vi "10-Tap 8-bit Camera without DRAM (FPGA-SIM)RandomSimDataNoHostDMAsNoAnalysis.vi"() -> ()   [LabVIEW 2013]
doc: "This is the FPGA VI for the 10-Tap 8-Bit Camera with DRAM example. This example demonstrates how to acquire images from a 10-tap, 8-bit, extended configuration, Camera Link camera and transfer the images to the host. This example supports area scan and line scan cameras for both continuous and finite acquisitions.\n\nThis example also demonstrates the use of DRAM as a frame buffer for very high speed acquisitions. Data packing and flow-control are also employed to maximize use of the available DRAM and FIFOs in terms of both memory space and performance.\n\nAdditionally, the example demonstrates the serial server, which allows third-party camera configuration utilities to communicate with the camera using the Camera Link serial interface while this VI is running."
uses:
  <vilib>/rvi/DataTransferAndStorage/Container/XNode/niFpgaContainer.xnode
  <vilib>/Platform/TimedLoop/XDataNode/XDataNode.xnode
  <vilib>/Platform/TimedLoop/XDataNode/timing_clust.ctl
  <vilib>/Platform/TimedLoop/XDataNode/XDNodeRunTimeDep.lvlib
  <vilib>/Platform/TimedLoop/XDataNode/wakeup.ctl
  <vilib>/Platform/TimedLoop/XDataNode/nitl_modes.ctl
  <vilib>/rvi/FIFO/Fifo_Resource/nirvififoEmulationRead.vi
  <vilib>/rvi/FIFO/Fifo_Resource/nirvififoEmulationWrite.vi
  FPGA/Globals/Accumulated Sector Intensity.vi
  FPGA/Globals/Pixel Location Global.vi
  FPGA/Globals/Wing Square Wave Frequency Global.vi
  FPGA/Globals/Sector Parameter Global.vi
  <vilib>/rvi/FIFO/Fifo_Resource/nirvififoEmulationGetNumberOfElementsToWrite.vi
  <vilib>/rvi/FIFO/Fifo_Resource/nirvififoEmulationGetNumberOfElementsToRead.vi
  Common/CL Signal Mapping.ctl
  Common/CL Configuration.ctl
  FPGA/Sector/Accumulate/Sector Parameter Cluster.ctl
panel:
  in  "Sim Data":u64=44
  out "Number of Elements to Write Sector Grouping FIFO":u32
  out "Accumulate Ticks":u32
  out "Analysis Ticks":u32
  out "Target Sim TO":bool
  out "Cam Data Timeout":bool
  out "Sector FIFO Timeout":bool
  out "Host DMA Timeout":bool
  out "Number of Elements to Read Cam Data":u32
  out "Number of Elements to Write Host DMA":u32
  in  "Words per image":u32=1000
  in  "Y Resolution":u16=1000
  in  "X Resolution":u16=1000
  in  "[Average BG Intensity]":u8[](array[numeric])=[0, 0, 0, 0, 0, 0, 0, 0, 0, 0, 0, 0, 0, 0, 0, 0, 0, 0, 0, 0, 0, 0, 0, 0, 0, 0, 0, 0, 0, 0, 0, 0]
  in  "Sector Threshold":u8
  in  "# of Frames to Average":u8=1
  in  "Sector Parameters Right":T1={"Start Angle"=0.0, "End Angle"=0.4708251953125, "Inner Radius"=309, "Outter Radius"=405, "Hinge X"=685, "Hinge Y"=527, "NumWingSectors"=8}
  in  "Sector Parameters Left":T1={"Start Angle"=0.65740966796875, "End Angle"=0.99468994140625, "Inner Radius"=309, "Outter Radius"=405, "Hinge X"=464, "Hinge Y"=534, "NumWingSectors"=8}
  in  "CL Config.Configuration":T2=enum."Full"
  in  "CL Config.Signal Mapping":T3=enum."Basler 10-tap"
  in  "CL Config.Line Scan":bool
  in  "CL Config.DVAL Active High":bool=TRUE
  in  "CL Config.LVAL Active High":bool=TRUE
  in  "CL Config.FVAL Active High":bool=TRUE
  in  "CL Config.Spare Active High":bool=TRUE
  in  "Acq Control.Line Scan Height":u32
  in  "Acq Control.Frames To Acq":u32
  in  "Acq Control.Acquire":bool
  in  "Acq Control.Cancel Acq":bool
  in  "Acq Control.Ignore DVAL":bool
  in  "Acq Control.Initialize":bool
  out "Acq Status.Acq In Progress":bool
  out "Acq Status.Clocks Per Line":u32
  out "Acq Status.Frames Acq'd":u32
  out "Acq Status.Lines Per Frame":u32
  out "Acq Status.DMA Write Timeout":bool
  out "Acq Status.Initialized":bool
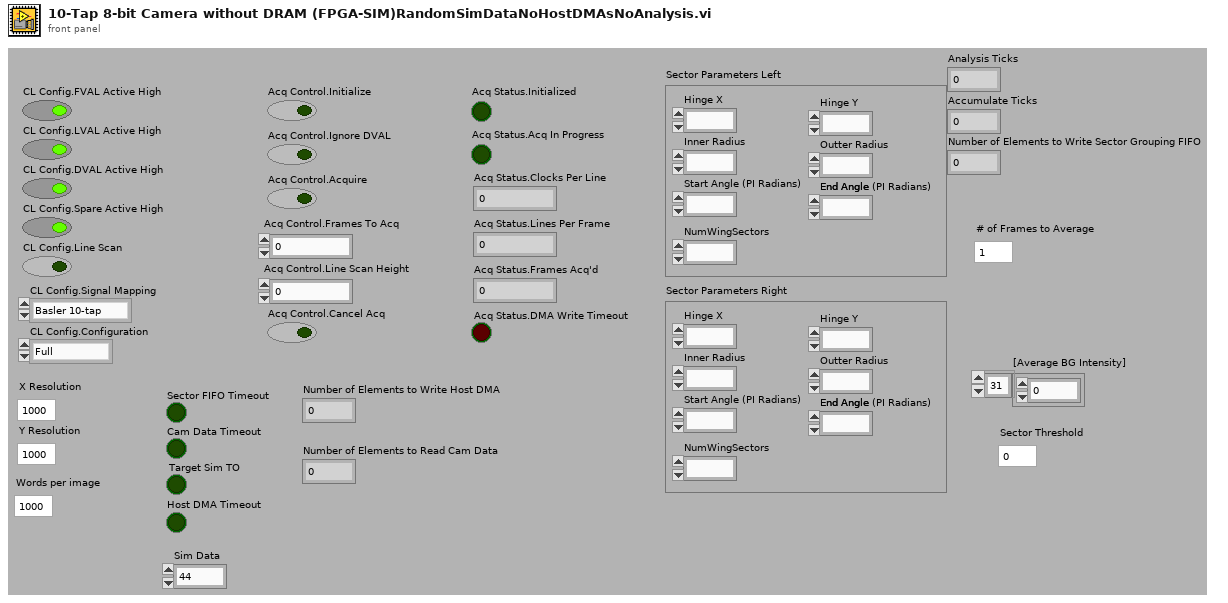
[diagram p1: front panel]
types:
  T1 = typedef "Sector Parameter Cluster.ctl" = cluster{"Start Angle":fxp<+/-,17,2>, "End Angle":fxp<+,17,3>, "Inner Radius":u16, "Outter Radius":u16, "Hinge X":u16, "Hinge Y":u16, "NumWingSectors":u8}
  T2 = typedef "CL Configuration.ctl" = enum8{"Base", "Medium", "Full"}
  T3 = typedef "CL Signal Mapping.ctl" = enum8{"Standard", "Basler 10-tap", "Vosskühler 10-tap"}
  T4 = typedef "XDNodeRunTimeDep.lvlib/timing_clust.ctl" = cluster{"Expected End [f-1]":u64, "Actual End [f-1]":u64, "Finished Late? [f-1]":bool, "Expected End [i-1]":u64, "Actual End [i-1]":u64, "Finished Late? [i-1]":bool, "Expected Start [i]":u64, "Actual Start [i]":u64, "Expected Start [f]":u64, "Actual Start [f]":u64, "Source Name":string, "Structure Name":string, "Period":i64, "Deadline":i64, "Offset":i64, "Start":i64, "Priority":i32, "Timeout":i32, "Mode":T5, "Wakeup Reason":T6, "Error":errorcluster, "Source Type":string, "Secondary Source Type":string, "Global End Time":u64, "Global Start Time":u64, "Frame Duration":u64, "Iteration Duration":u64, "Assigned CPU":i32, "I/O Scan Engine Mode":u32}
  T5 = typedef "XDNodeRunTimeDep.lvlib/nitl_modes.ctl" = enum32{"No Change", "Process missed periods, maintain original phase", "Discard missed periods, maintain original phase", "Process missed periods, ignore original phase", "Discard missed periods, ignore original phase"}
  T6 = typedef "XDNodeRunTimeDep.lvlib/wakeup.ctl" = enum32{"Normal", "Aborted", "Asynchronous wakeup", "Timing source error", "Timed loop error", "Timeout"}
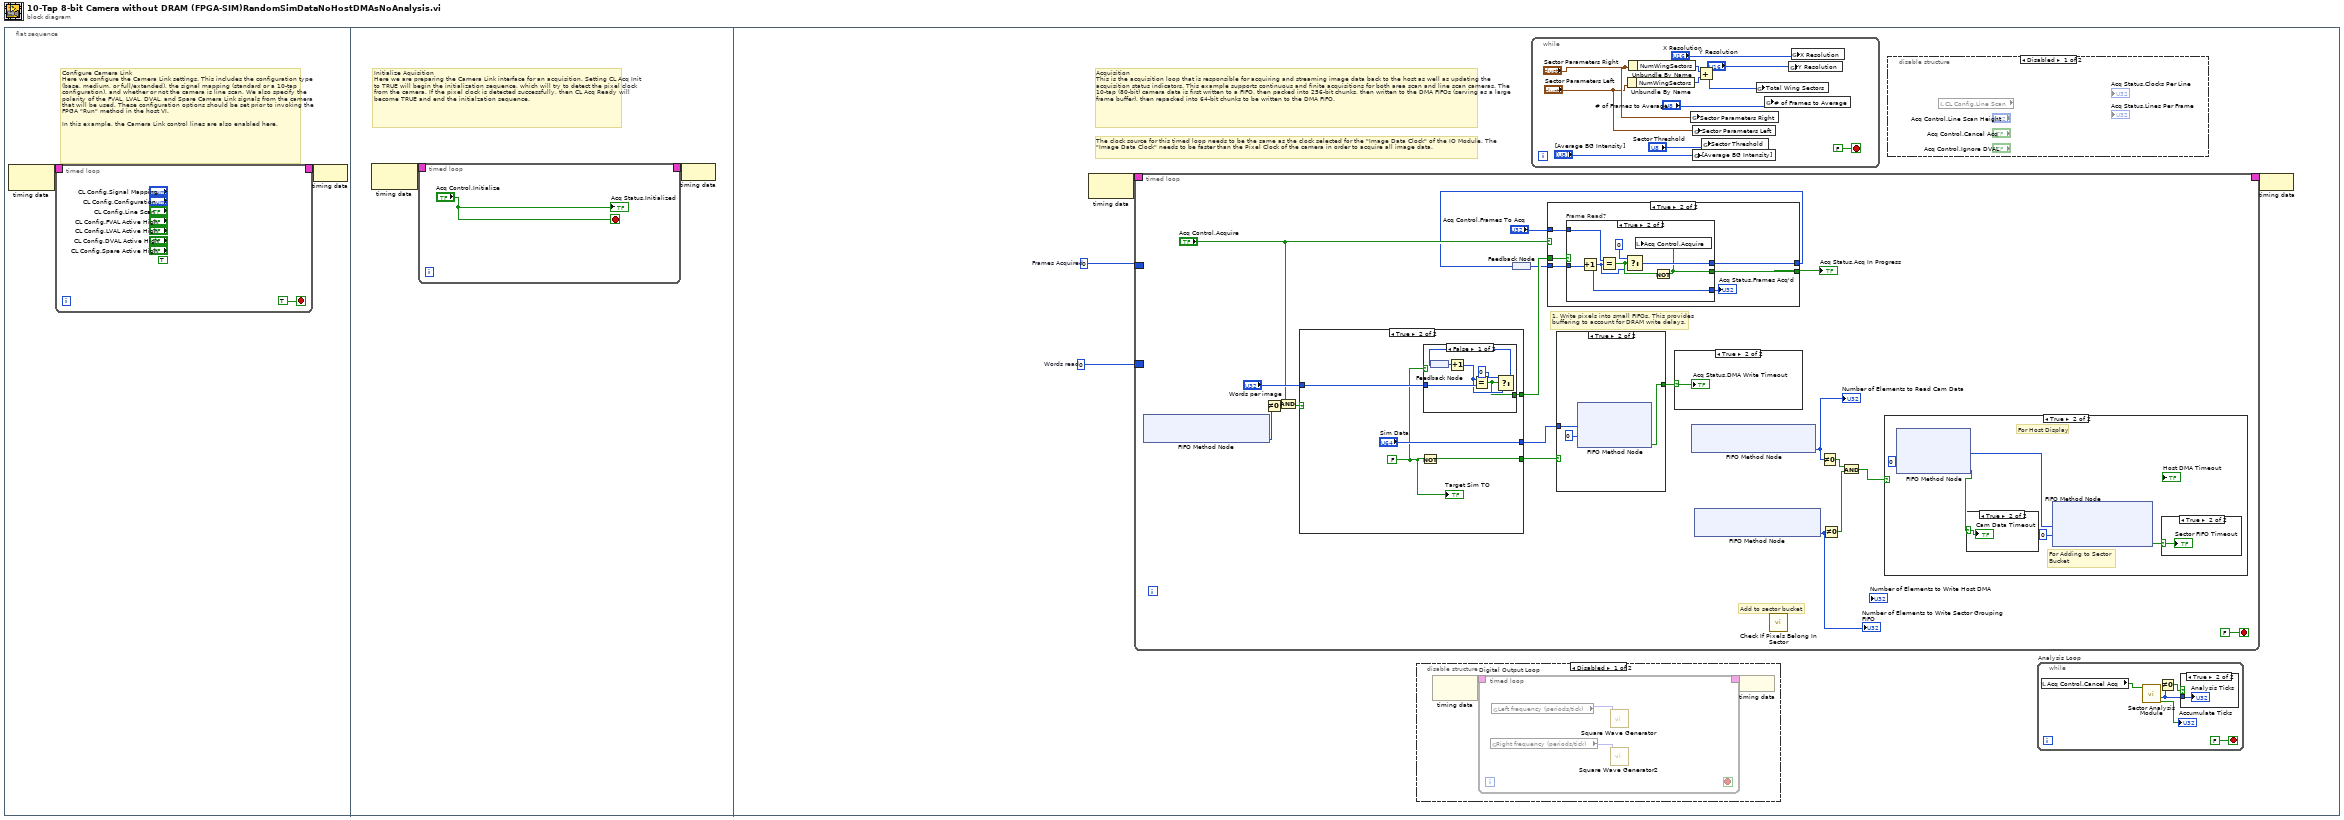
[diagram p0: block diagram]
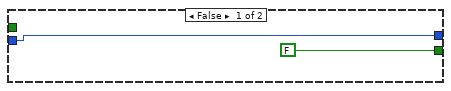
[diagram p6: hidden frame]
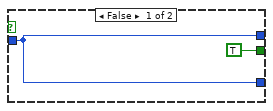
[diagram p7: hidden frame]
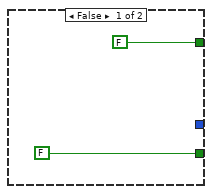
[diagram p8: hidden frame]
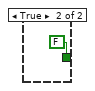
[diagram p9: hidden frame]
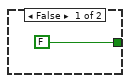
[diagram p13: hidden frame]
diagram:
  n1 = flat-sequence {
    frame #0 {
      # "Configure Camera Link\nHere we configure the Camera Link settings. This includes the configuration type (base, medium, or full/extended), the signal mapping (standard or a 10-tap configuration), and whether or not the camera is line scan. We also specify the polarity of the FVAL, LVAL, DVAL, and Spare Camera Link signals from the camera that will be used. These configuration options should be set prior to invoking the FPGA \"Run\" method in the host VI.\n\nIn this example, the Camera Link control lines are also enabled here."
      n2 = node-c288() -> (w2:T4)  [unwired: 1 in]
      n3 = timed-loop {
        timing: w2 -> [_]
        timing-out: [_] -> w1
        stop <- TRUE stop-if-true
        (unwired) TRUE ("IO Module\\CL Control Enable")
      }
      n4 = node-c288(w1) -> ()
    }
    frame #1 {
      # "Initialize Aquisition\nHere we are preparing the Camera Link interface for an acquisition. Setting CL Acq Init to TRUE will begin the initialization sequence, which will try to detect the pixel clock from the camera. If the pixel clock is detected successfully, then CL Acq Ready will become TRUE and end the initialzation sequence."
      n5 = node-c288() -> (w9:T4)  [unwired: 1 out]
      n6 = timed-loop {
        timing: w9 -> [_]
        timing-out: [_] -> w8
        stop <- "Acq Control.Initialize" stop-if-true
        "Acq Status.Initialized" <- "Acq Control.Initialize"
      }
      n7 = node-c288(w8) -> ()
    }
    frame #2 {
      w15 = u32 0  # Frames Acquired
      w16 = u32 0  # Words read
      # "The clock source for this timed loop needs to be the same as the clock selected for the \"Image Data Clock\" of the IO Module. The \"Image Data Clock\" needs to be faster than the Pixel Clock of the camera in order to acquire all image data."
      # "Acquisition\nThis is the acquisition loop that is responsible for acquiring and streaming image data back to the host as well as updating the acquisition status indicators. This example supports continuous and finite acquisitions for both area scan and line scan cameras. The 10-tap (80-bit) camera data is first written to a FIFO, then packed into 256-bit chunks, then written to the DMA FIFOs (serving as a large frame buffer), then repacked into 64-bit chunks to be written to the DMA FIFO."
      n8 = node-c288() -> (w18:T4)  [unwired: 1 in]
      n9 = timed-loop {
        timing: w18 -> [_]
        timing-out: [_] -> w17
        border: w16 -> [_]
        border: w15 -> [_]
        stop <- FALSE stop-if-true
        # "Add to sector bucket"
        # "1. Write pixels into small FIFOs. This provides\nbuffering to account for DRAM write delays."
        n10 = xnode ("FIFO Method Node")() -> ("Number of Elements to Write"=w47:u32)  [unwired: 1 in, 1 out]
        n11 = Not Equal To 0?(x=w47) -> (x != 0?=w46:bool)
        n12 = Compound Arithmetic op=AND("Acq Control.Acquire", w46) -> (w52:bool)
        n13 = case shown="True" w52 {
          tunnel: [_ "Sim Data"] -> w56
          tunnel: [FALSE w79] -> w54
          tunnel: "Words per image" -> [_ w81]
          tunnel: [FALSE w80] -> w43
          frame False {
          }
          frame True {
            w77 = FALSE ("x")
            n14 = Not(x=w77) -> (.not. x?=w79:bool)
            n15 = case shown="False" w77 {
              tunnel: w81 -> [w87 _]
              tunnel: [w82 FALSE] -> w80
              frame False {
                n16 = feedback #1() -> (w86:u32)
                n17 = Increment(x=w86) -> (x+1=w83:u32)
                n18 = Equal?(x=w83, y=w87) -> (x = y?=w82:bool)
                n19 = Select(t=u32 0 ("Acq Status.Frames Acq'd"), s=w82, f=w83) -> (s? t:f=w84:u32)
                n20 = feedback-in #1(w84) -> ()
              }
              frame True {
              }
            }
            "Target Sim TO" <- w77
          }
        }
        n21 = feedback #2() -> (w42:u32)
        n22 = case shown="True" "Acq Control.Acquire" {
          tunnel: w43 -> [_ w65]
          tunnel: w42 -> [w59 w64]
          tunnel: "Acq Control.Frames To Acq" -> [_ w63]
          tunnel: [w59 w62] -> w40
          tunnel: [FALSE w61] -> w39
          frame False {
          }
          frame True {
            n23 = case "Frame Read?" shown="True" w65 {
              tunnel: w64 -> [w66 w74]
              tunnel: w63 -> [_ w73]
              tunnel: [w66 w71] -> w62
              tunnel: [TRUE w69] -> w61
              tunnel: [w66 w68] -> w60
              frame False {
              }
              frame True {
                n24 = Increment(x=w74) -> (x+1=w68:u32)
                n25 = Equal?(x=w73, y=w68) -> (x = y?=w70:bool)
                n26 = Select(t=u32 0 ("Frames Acquired"), s=w70, f=w68) -> (s? t:f=w71:u32)
                n27 = Not(x=w70) -> (.not. x?=w69:bool)
                n28 = local write "Acq Control.Acquire"(w69) -> ()
              }
            }
            "Acq Status.Frames Acq'd" <- w60
          }
        }
        "Acq Status.Acq In Progress" <- w39
        n29 = feedback-in #2(w40) -> ()
        n30 = case shown="True" w54 {
          tunnel: [FALSE ("Timed Out?") w98] -> w38
          tunnel: w56 -> [_ w99]
          frame False {
          }
          frame True {
            n31 = xnode ("FIFO Method Node")("Element"=w99, "Timeout"=0) -> ("Timed Out?"=w98:bool)  [unwired: 1 in, 1 out]
          }
        }
        n32 = case shown="True" w38 {
          selector: w38 -> [_ w57]
          frame False {
          }
          frame True {
            "Acq Status.DMA Write Timeout" <- w57
          }
        }
        n33 = xnode ("FIFO Method Node")() -> ("Number of Elements to Read"=w49:u32)  [unwired: 1 in, 1 out]
        "Number of Elements to Read Cam Data" <- w49
        n34 = xnode ("FIFO Method Node")() -> ("Number of Elements to Write"=w51:u32)  [unwired: 1 in, 1 out]
        "Number of Elements to Write Sector Grouping FIFO" <- w51
        n35 = call "Check If Pixels Belong In Sector.vi"() -> ()  [unwired: 11 in, 1 out]
        n36 = Not Equal To 0?(x=w49) -> (x != 0?=w48:bool)
        n37 = Not Equal To 0?(x=w51) -> (x != 0?=w50:bool)
        n38 = Compound Arithmetic op=AND(w48, w50) -> (w53:bool)
        n39 = case shown="True" w53 {
          frame False {
          }
          frame True {
            # "For Adding to Sector \nBucket"
            # "For Host Display"
            n40 = xnode ("FIFO Method Node")("Timeout"=0) -> ("Element"=w92:u64, "Timed Out?"=w89:bool)  [unwired: 1 in, 1 out]
            n41 = case shown="True" w89 {
              selector: w89 -> [_ w94]
              frame False {
              }
              frame True {
                "Cam Data Timeout" <- w94
              }
            }
            n42 = xnode ("FIFO Method Node")("Element"=w92, "Timeout"=0) -> ("Timed Out?"=w90:bool)  [unwired: 1 in, 1 out]
            n43 = case shown="True" w90 {
              selector: w90 -> [_ w95]
              frame False {
              }
              frame True {
                "Sector FIFO Timeout" <- w95
              }
            }
          }
        }
      }
      n44 = disable-structure shown="Disabled" {
        frame Disabled {
          n45 = node-c288() -> (w25:T4)  [unwired: 1 in]
          n46 = timed-loop "Digital Output Loop" {
            timing: w25 -> [_]
            timing-out: [_] -> w24
            stop <- _ stop-if-true
            n47 = global read "Wing Square Wave Frequency Global.vi" "Right frequency (periods/tick)"() -> (w26:fxp<+,32,0>)
            n48 = global read "Wing Square Wave Frequency Global.vi" "Left frequency (periods/tick)"() -> (w27:fxp<+,32,0>)
            n49 = call "Square Wave Generator"("frequency (periods/tick)"=w27) -> ()  [unwired: 14 in, 1 out]
            n50 = call "Square Wave Generator2"("frequency (periods/tick)"=w26) -> ()  [unwired: 14 in, 1 out]
          }
          n51 = node-c288(w24) -> ()
        }
        frame Enabled {
        }
      }
      n52 = while {
        stop <- FALSE stop-if-true
        n53 = Unbundle By Name("Sector Parameters Left") -> ("NumWingSectors"=w112:u8)
        n54 = Unbundle By Name("Sector Parameters Right") -> ("NumWingSectors"=w113:u8)
        n55 = global write "Sector Parameter Global.vi" "Sector Parameters Right"("Sector Parameters Right") -> ()
        n56 = global write "Sector Parameter Global.vi" "Sector Parameters Left"("Sector Parameters Left") -> ()
        n57 = global write "Sector Parameter Global.vi" "[Average BG Intensity]"("[Average BG Intensity]") -> ()
        n58 = Add(x=w113, y=w112) -> (x+y=w111:u8)
        n59 = global write "Sector Parameter Global.vi" "Sector Threshold"("Sector Threshold") -> ()
        n60 = global write "Accumulated Sector Intensity.vi" "Total Wing Sectors"(w111) -> ()
        n61 = global write "Pixel Location Global.vi" "# of Frames to Average"("# of Frames to Average") -> ()
        n62 = global write "Pixel Location Global.vi" "Y Resolution"("Y Resolution") -> ()
        n63 = global write "Pixel Location Global.vi" "X Resolution"("X Resolution") -> ()
      }
      n64 = disable-structure shown="Disabled" {
        frame Disabled {
          n65 = local read "CL Config.Line Scan"() -> (w21:bool)
        }
        frame Enabled {
        }
      }
      n66 = while "Analysis Loop" {
        stop <- FALSE stop-if-true
        n67 = local read "Acq Control.Cancel Acq"() -> (w35:bool)
        n68 = call "Sector Analysis Module.vi"("Canceled?"=w35) -> ("New Data? Out"=→"Accumulate Ticks":bool, "Analysis Ticks"=w33:u32)  [unwired: 6 in, 3 out]
        n69 = Not Equal To 0?(x=w33) -> (x != 0?=w32:bool)
        n70 = case shown="True" w32 {
          tunnel: w33 -> [_ w37]
          frame False {
          }
          frame True {
            "Analysis Ticks" <- w37
          }
        }
      }
      n71 = node-c288(w17) -> ()
    }
  }
